vi "UEGO.vi"(8 "error in (no error)":errorcluster, 11 "Node Ptr":T2 format="%.0x") -> (0 "error out":errorcluster)   [LabVIEW 2016, in "DCM System Explorer.lvlib"]
uses:
  DCM System Explorer.lvlib
  <vilib>/NI Veristand/Custom Device API/Custom Device Item Ref.ctl
  Shared/DCM Constants and GUIDs.vi
  <vilib>/NI Veristand/Custom Device Tools/Custom Device Utility Library/NI VeriStand - Search for Item by Name.vi
  <vilib>/NI VeriStand/Custom Device API/Custom Device API.lvlib
  DCM Shared.lvlib
  <vilib>/NI Veristand/Custom Device Tools/Custom Device Utility Library/Custom Device Utility Library.lvlib
panel:
  in  "SensorControl":T1={"UEGO1Enable"=FALSE, "UEGO2Enable"=FALSE, "UEGO1Range"=FALSE, "UEGO2Range"=FALSE, "FilterCutoff (Hz)"=10.0}
  in  "Header":cluster{"Section Name":string}={"Section Name"="UEGO Initial Settings"}
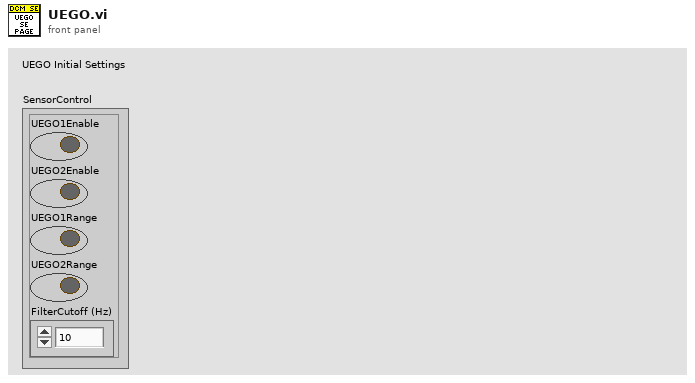
[diagram p1: front panel]
types:
  T1 = cluster{"UEGO1Enable":bool, "UEGO2Enable":bool, "UEGO1Range":bool, "UEGO2Range":bool, "FilterCutoff (Hz)":dbl}
  T2 = typedef "Custom Device API.lvlib/Custom Device Item Ref.ctl" = u64
  T3 = typedef "DCM Shared.lvlib/Channel.ctl" = cluster{"Name":string, "Units":string, "Default":dbl, "Description":string}
  T4 = typedef "Custom Device API.lvlib/Custom Device Channel.ctl" = cluster{"Type":T5, "Units":string, "Default Value":dbl, "Faultable":bool, "Scalable":bool}
  T5 = typedef "Custom Device API.lvlib/Custom Device Channel Type.ctl" = enum16{"Input", "Output"}
  T6 = typedef "Custom Device API.lvlib/Custom Device Commands.ctl" = enum16{"Default", "Item renamed", "Shutdown", "Dynamic button pressed"}
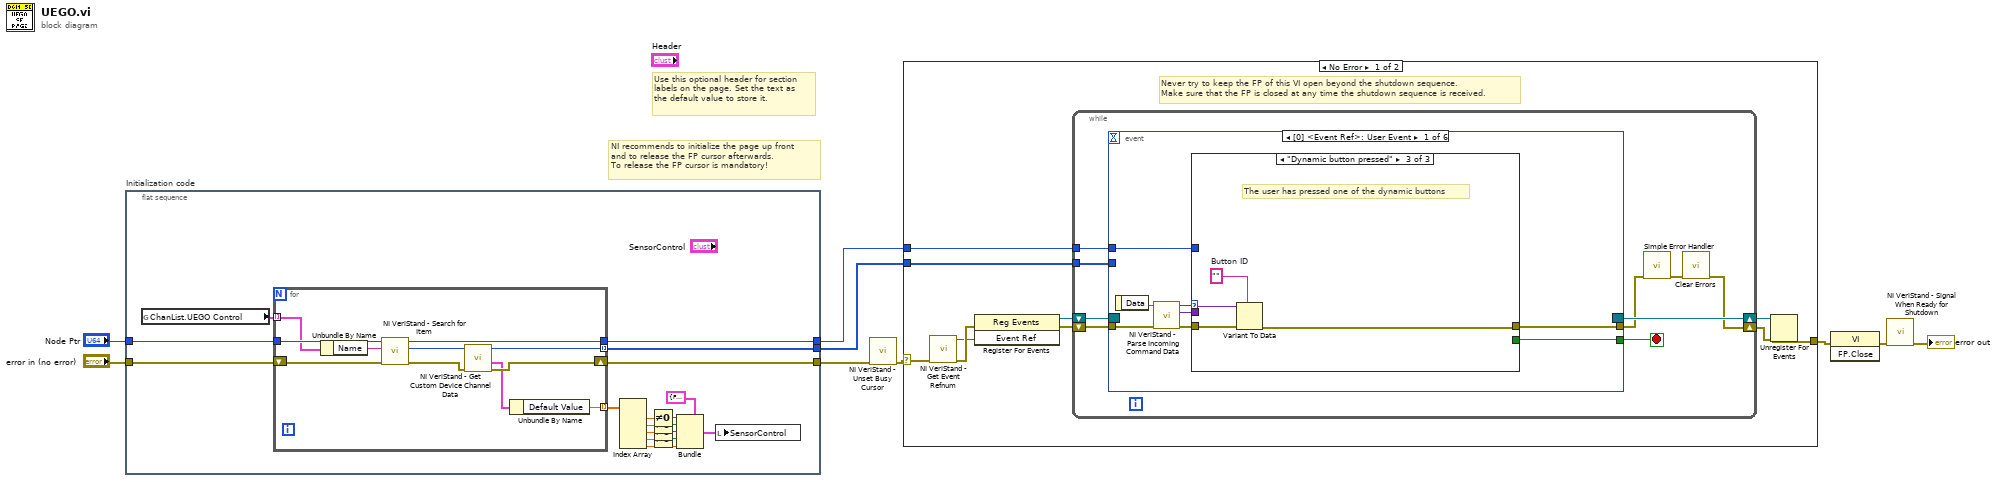
[diagram p0: block diagram]
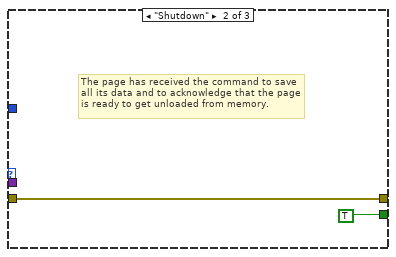
[diagram p3: hidden frame]
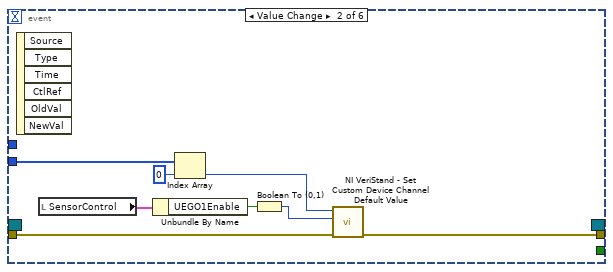
[diagram p4: hidden frame]
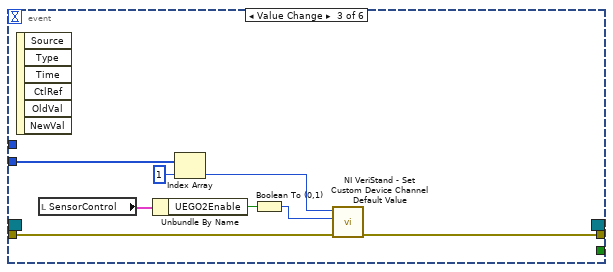
[diagram p5: hidden frame]
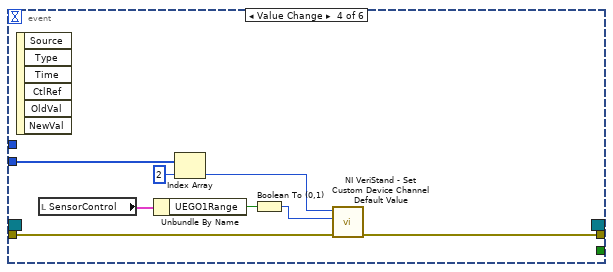
[diagram p6: hidden frame]
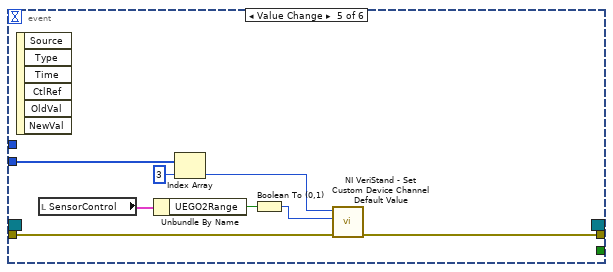
[diagram p7: hidden frame]
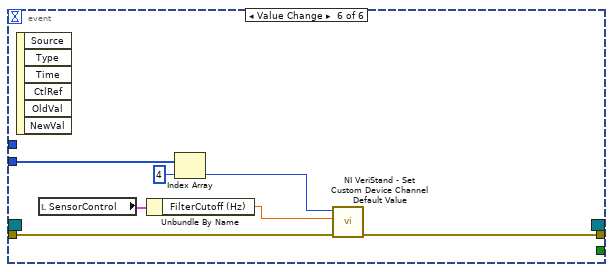
[diagram p8: hidden frame]
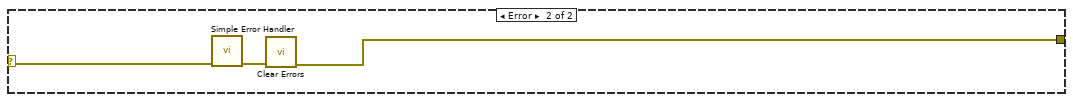
[diagram p9: hidden frame]
diagram:
  # "Use this optional header for section labels on the page. Set the text as the default value to store it."
  # "NI recommends to initialize the page up front\nand to release the FP cursor afterwards.\nTo release the FP cursor is mandatory!"
  n1 = flat-sequence "Initialization code" {
    tunnel: [w27] -> w2
    tunnel: [w26] -> w5
    tunnel: "Node Ptr" -> [w23]
    tunnel: "error in (no error)" -> [w22]
    tunnel: [w10] -> w1
    frame #0 {
      n2 = global read "DCM Constants and GUIDs.vi" "ChanList.UEGO Control"() -> (w24:T3[])
      n3 = for {
        tunnel: w23 -> [w38]
        tunnel: [w36] -> w27
        shift-right: [w31] -> w26
        shift-left: w22 -> [w37]
        tunnel: w24 -> [w35] mode=indexing
        tunnel: [w29] -> w25 mode=indexing
        tunnel: [w28] -> w10 mode=indexing
        n4 = Unbundle By Name(w35) -> ("Name"=w34:string)
        n5 = call-poly <vilib>:"NI VeriStand - Search for Item.vi"("error in"=w37, "Item Name"=w34, "Section Ref in"=w38) -> ("error out"=w33:errorcluster, "Item Ref"=w32:T2, "Section Ref out"=w36:T2)  [unwired: 5 in, 1 out]
        n6 = call <vilib>:"NI VeriStand - Get Custom Device Channel Data.vi"("error in (no error)"=w33, "Channel Ref in"=w32) -> ("error out"=w31:errorcluster, "Channel"=w30:T4, "Channel Ref out"=w28:T2)  [unwired: 4 in, 3 out]
        n7 = Unbundle By Name(w30) -> ("Default Value"=w29:dbl)
      }
      n8 = Index Array(array=w25) -> (element #1=w19:dbl, element #2=w18:dbl, element #3=w17:dbl, element #4=w16:dbl, element #5=w11:dbl)  [unwired: 5 in]
      n9 = Not Equal To 0?(x=w19) -> (x != 0?=w15:bool)
      n10 = Not Equal To 0?(x=w18) -> (x != 0?=w14:bool)
      n11 = Not Equal To 0?(x=w17) -> (x != 0?=w13:bool)
      n12 = Not Equal To 0?(x=w16) -> (x != 0?=w12:bool)
      n13 = Bundle(cluster=T1 {"UEGO1Enable"=FALSE, "UEGO2Enable"=FALSE, "UEGO1Range"=FALSE, "UEGO2Range"=FALSE, "FilterCutoff (Hz)"=10.0} ("SensorControl"), "UEGO1Enable"=w15, "UEGO2Enable"=w14, "UEGO1Range"=w13, "UEGO2Range"=w12, "FilterCutoff (Hz)"=w11) -> (w20:T1)
      n14 = local write "SensorControl"(w20) -> ()
    }
  }
  n15 = call <vilib>:"NI VeriStand - Unset Busy Cursor.vi"("error in (no error)"=w5) -> ("error out"=w4:errorcluster)  [unwired: 10 out]
  n16 = case shown="No Error" w4 {
    selector: w4 -> [w40 w114]
    tunnel: [w45 w112] -> w9
    tunnel: w2 -> [w41 _]
    tunnel: w1 -> [w39 _]
    frame No Error {
      # "Never try to keep the FP of this VI open beyond the shutdown sequence.\nMake sure that the FP is closed at any time the shutdown sequence is received."
      n17 = call <vilib>:"NI VeriStand - Get Event Refnum.vi"("error in (no error)"=w40) -> ("error out"=w48:errorcluster, "Event Ref"=w44:refnum<user-event>)  [unwired: 9 out]
      n18 = register-events(error in=w48, w44) -> (reference out=w42:refnum<event-registration>, error out=w43:errorcluster)  [unwired: 1 in]
      n19 = while {
        tunnel: w41 -> [w53]
        shift-right: [w50] -> w46
        shift-left: w43 -> [w56]
        shift-right: [w57] -> w47
        shift-left: w42 -> [w55]
        tunnel: w39 -> [w49]
        stop <- w54 stop-if-true
        n20 = event shown="[0] <Event Ref>: User Event" {
          selector: w55 -> [_ _ _ _ _ _]
          dyn-events: [_ _ _ _ _ _] -> w57
          timeout: _ -> [_ _ _ _ _ _]
          tunnel: w56 -> [w65 w80 w88 w96 w104 w111]
          tunnel: [w61 _ _ _ _ _] -> w54
          tunnel: [w60 w79 w87 w95 w103 w110] -> w52
          tunnel: w53 -> [w59 _ _ _ _ _]
          tunnel: w49 -> [_ w78 w86 w94 w102 w109]
          event User Event {
            n21 = event-data() -> ("Data"=w64:string)  [unwired: 1 out]
            n22 = call <vilib>:"NI VeriStand - Parse Incoming Command Data.vi"("error in (no error)"=w65, "Incoming data"=w64) -> ("error out"=w63:errorcluster, "Outgoing data"=w58:variant, "Action"=w62:T6)  [unwired: 7 out]
            n23 = case shown="\"Dynamic button pressed\"" w62 {
              tunnel: w63 -> [w66 w67 w72]
              tunnel: [_ TRUE _] -> w61
              tunnel: [w66 w67 w69] -> w60
              tunnel: w59 -> [_ _ _]
              tunnel: w58 -> [_ _ w71]
              frame "Default", Default {
              }
              frame "Shutdown" {
                # "The page has received the command to save all its data and to acknowledge that the page is ready to get unloaded from memory."
              }
              frame "Dynamic button pressed" {
                w70 = ""  # Button ID
                # "The user has pressed one of the dynamic buttons"
                n24 = Variant To Data(error in=w72, type=w70, Variant=w71) -> (error out=w69:errorcluster)  [unwired: 1 out]
              }
            }
          }
          event "SensorControl.UEGO1Enable": Value Change {
            n25 = event-data() -> ()  [unwired: 7 out]
            n26 = local read "SensorControl"() -> (w76:T1)
            n27 = Unbundle By Name(w76) -> ("UEGO1Enable"=w75:bool)
            n28 = Index Array(array=w78, index=0) -> (element=w77:T2)
            n29 = Boolean To (0,1)(Boolean=w75) -> (0, 1=w74:i16)
            n30 = call <vilib>:"NI VeriStand - Set Custom Device Channel Default Value.vi"("error in (no error)"=w80, "Default Value"=w74, "Channel Ref in"=w77) -> ("error out"=w79:errorcluster)  [unwired: 7 in, 1 out]
          }
          event "SensorControl.UEGO2Enable": Value Change {
            n31 = event-data() -> ()  [unwired: 7 out]
            n32 = local read "SensorControl"() -> (w84:T1)
            n33 = Unbundle By Name(w84) -> ("UEGO2Enable"=w83:bool)
            n34 = Index Array(array=w86, index=1) -> (element=w85:T2)
            n35 = Boolean To (0,1)(Boolean=w83) -> (0, 1=w82:i16)
            n36 = call <vilib>:"NI VeriStand - Set Custom Device Channel Default Value.vi"("error in (no error)"=w88, "Default Value"=w82, "Channel Ref in"=w85) -> ("error out"=w87:errorcluster)  [unwired: 7 in, 1 out]
          }
          event "SensorControl.UEGO1Range": Value Change {
            n37 = event-data() -> ()  [unwired: 7 out]
            n38 = local read "SensorControl"() -> (w92:T1)
            n39 = Unbundle By Name(w92) -> ("UEGO1Range"=w91:bool)
            n40 = Index Array(array=w94, index=2) -> (element=w93:T2)
            n41 = Boolean To (0,1)(Boolean=w91) -> (0, 1=w90:i16)
            n42 = call <vilib>:"NI VeriStand - Set Custom Device Channel Default Value.vi"("error in (no error)"=w96, "Default Value"=w90, "Channel Ref in"=w93) -> ("error out"=w95:errorcluster)  [unwired: 7 in, 1 out]
          }
          event "SensorControl.UEGO2Range": Value Change {
            n43 = event-data() -> ()  [unwired: 7 out]
            n44 = local read "SensorControl"() -> (w100:T1)
            n45 = Unbundle By Name(w100) -> ("UEGO2Range"=w99:bool)
            n46 = Index Array(array=w102, index=3) -> (element=w101:T2)
            n47 = Boolean To (0,1)(Boolean=w99) -> (0, 1=w98:i16)
            n48 = call <vilib>:"NI VeriStand - Set Custom Device Channel Default Value.vi"("error in (no error)"=w104, "Default Value"=w98, "Channel Ref in"=w101) -> ("error out"=w103:errorcluster)  [unwired: 7 in, 1 out]
          }
          event "SensorControl.FilterCutoff (Hz)": Value Change {
            n49 = event-data() -> ()  [unwired: 7 out]
            n50 = local read "SensorControl"() -> (w107:T1)
            n51 = Unbundle By Name(w107) -> ("FilterCutoff (Hz)"=w106:dbl)
            n52 = Index Array(array=w109, index=4) -> (element=w108:T2)
            n53 = call <vilib>:"NI VeriStand - Set Custom Device Channel Default Value.vi"("error in (no error)"=w111, "Default Value"=w106, "Channel Ref in"=w108) -> ("error out"=w110:errorcluster)  [unwired: 7 in, 1 out]
          }
        }
        n54 = call <vilib>:"Simple Error Handler.vi"("error in (no error)"=w52) -> ("error out"=w51:errorcluster)  [unwired: 1 in, 7 out]
        n55 = call <vilib>:"Clear Errors.vi"("error in (no error)"=w51) -> ("error out"=w50:errorcluster)  [unwired: 1 in, 5 out]
      }
      n56 = Unregister For Events(event registration refnum=w47, error in=w46) -> (error out=w45:errorcluster)
    }
    frame Error {
      n57 = call <vilib>:"Simple Error Handler.vi"("error in (no error)"=w114) -> ("error out"=w113:errorcluster)  [unwired: 1 in, 7 out]
      n58 = call <vilib>:"Clear Errors.vi"("error in (no error)"=w113) -> ("error out"=w112:errorcluster)  [unwired: 1 in, 5 out]
    }
  }
  n59 = invoke class="VI" method="FP.Close"(error in=w9) -> (error out=w8:errorcluster)  [unwired: 2 in, 2 out]
  n60 = call <vilib>:"NI VeriStand - Signal When Ready for Shutdown.vi"("error in (no error)"=w8) -> ("error out"=→"error out":errorcluster)  [unwired: 10 out]
